vi "Save Libary to Disk.vi"(5 "Library Name":string="Engine.lvlib", 7 "Target Name":string="My Computer", 8 "error in (no error)":errorcluster, 10 "Destination Directories":path[](array[path]), 11 "Project Sync Tools in":refnum<class "Project Sync Tools.lvclass">) -> (0 "error out":errorcluster, 2 "New Library Paths":path[](array[path]), 3 "Project Sync Tools out":refnum<class "Project Sync Tools.lvclass">)   [LabVIEW 2019, in "Project Sync Tools.lvclass"]
uses:
  Project Sync Tools.lvclass
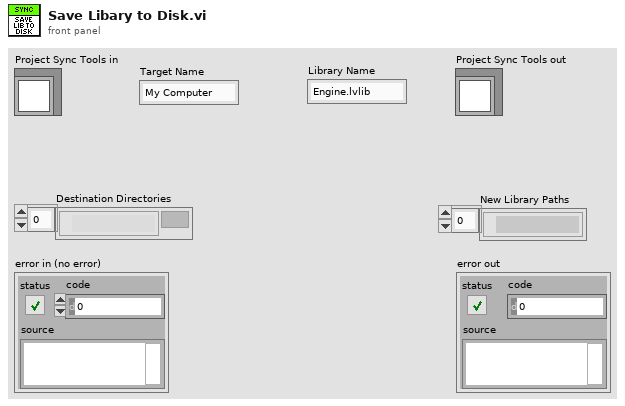
[diagram p1: front panel]
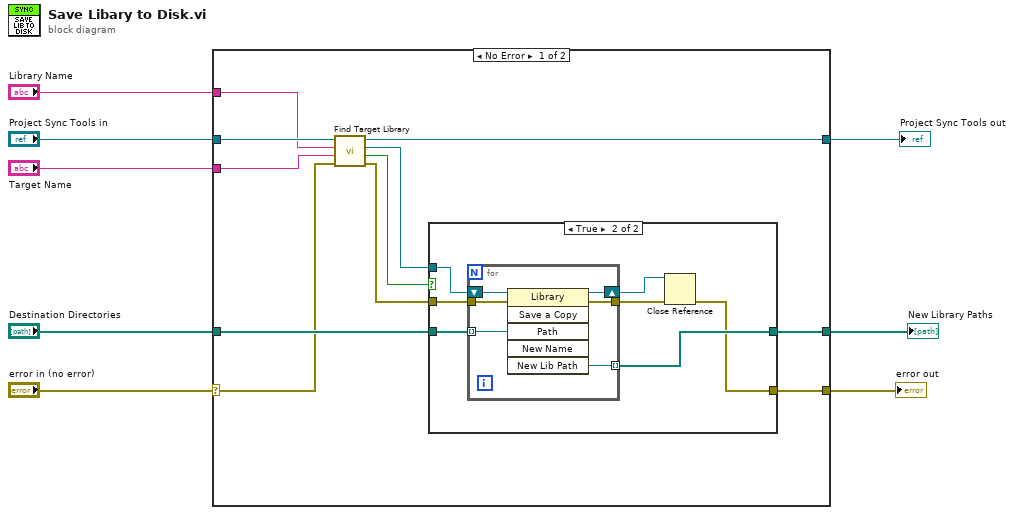
[diagram p0: block diagram]
diagram:
  n1 = case shown="No Error" "error in (no error)" {
    selector: "error in (no error)" -> [w14 w35]
    tunnel: [w18 w34] -> w8
    tunnel: "Destination Directories" -> [w17 _]
    tunnel: "Project Sync Tools in" -> [w16 w34]
    tunnel: [w12 w35] -> w5
    tunnel: [w15 _] -> w4
    tunnel: "Target Name" -> [w10 _]
    tunnel: "Library Name" -> [w9 _]
    frame No Error {
      n2 = call "Find Target Library.vi"("error in (no error)"=w14, "Target Name"=w10, "Library Name"=w9, "CD Build Tools in"=w16) -> ("error out"=w19:errorcluster, "Found ?"=w11:bool, "Library out"=w13:refnum<vi>, "CD Build Tools out"=w18:refnum<class "Project Sync Tools.lvclass">)  [unwired: 4 in]
      n3 = case shown="True" w11 {
        tunnel: w19 -> [w20 w27]
        tunnel: w17 -> [_ w26]
        tunnel: [_ w25] -> w15
        tunnel: w13 -> [_ w24]
        tunnel: [w20 w21] -> w12
        frame False {
        }
        frame True {
          n4 = for {
            tunnel: [w33] -> w23
            tunnel: w26 -> [w31] mode=indexing
            tunnel: w27 -> [w30]
            tunnel: [w29] -> w25 mode=indexing
            shift-right: [w28] -> w22
            shift-left: w24 -> [w32]
            n5 = invoke class="Library" method="Save a Copy"(reference=w32, error in=w30, "Path"=w31) -> (reference out=w28:refnum<vi>, error out=w33:errorcluster, "New Lib Path"=w29:path)  [unwired: 3 in, 3 out]
          }
          n6 = Close Reference(reference=w22, error in (no error)=w23) -> (error out=w21:errorcluster)
        }
      }
    }
    frame Error {
    }
  }
  "Project Sync Tools out" <- w8
  "error out" <- w5
  "New Library Paths" <- w4
